vi "Show Window Request.vi"(8 "error in (no error)":errorcluster, 11 "BuildWorker in":refnum<class "BuildWorker.lvclass">) -> (0 "error out":errorcluster, 3 "BuildWorker out":refnum<class "BuildWorker.lvclass">)   [LabVIEW 2017, in "BuildWorker.lvlib" / "BuildWorker.lvclass"]
uses:
  BuildWorker.lvclass
  <vilib>/ActorFramework/Actor/Actor.lvclass
  BuildWorker Messages/Send Worker Status Update Msg/Send Worker Status Update Msg.lvclass
  Framework/Actor wUI/Actor wUI.lvclass
  Volumes/Data/Users/benji667/Git/BuildFarm/src/LabVIEW/vi.lib/BenjaminR/Build Farm/Actors/Framework/Actor wUI/Actor wUI.lvclass
  Applications/National Instruments/LabVIEW 2017 64-bit/vi.lib/ActorFramework/Actor/Actor.lvclass
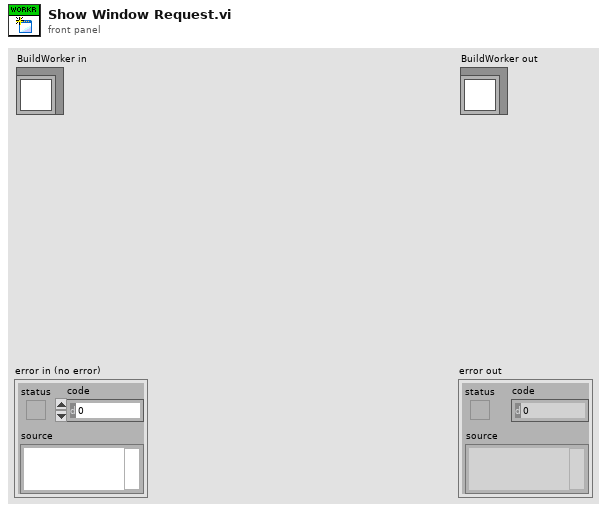
[diagram p1: front panel]
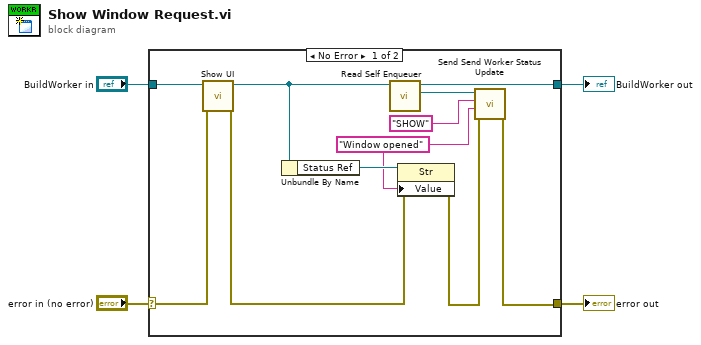
[diagram p0: block diagram]
diagram:
  n1 = case shown="No Error" "error in (no error)" {
    selector: "error in (no error)" -> [w6 w16]
    tunnel: [w10 w16] -> w3
    tunnel: [w7 w15] -> w1
    tunnel: "BuildWorker in" -> [w8 w15]
    frame No Error {
      w9 = "Window opened" ("Value")
      n2 = call "Show UI.vi"("error in (no error)"=w6, "Actor wUI in"=w8) -> ("error out"=w5:errorcluster, "Actor wUI out"=w7:refnum<class "BuildWorker.lvclass">)  [unwired: 8 in]
      n3 = Unbundle By Name(w7) -> ("Status Ref"=w14:refnum<vi>)
      n4 = call <vilib>:"Read Self Enqueuer.vi"("Actor"=w7) -> ("Self Enqueuer"=w13:refnum<class "Message Enqueuer.lvclass">)  [unwired: 10 in]
      n5 = property class="Str"(reference=w14, error in=w5, "Value"=w9) -> (error out=w11:errorcluster)  [unwired: 1 out]
      n6 = call "Send Send Worker Status Update.vi"("error in (no error)"=w11, "Status"=w9, "Operation"="SHOW", "Message Enqueuer in"=w13) -> ("error out"=w10:errorcluster)  [unwired: 6 in, 1 out]
    }
    frame Error {
    }
  }
  "error out" <- w3
  "BuildWorker out" <- w1
